vi "AlarmInsert.vi"(6 "提示":string="正常", 7 "takesTime":string, 9 "级别":string="10", 10 "类型":string="装配步骤", 11 "消息名":string) -> ()   [LabVIEW 2013]
uses:
  resultShow.vi
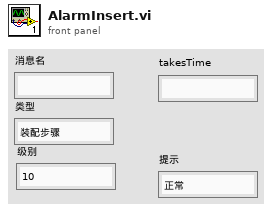
[diagram p1: front panel]
types:
  T1 = cluster{"takesTime":refnum<vi>, "userStatus":refnum<vi>, "userName":refnum<vi>, "connectionMode":refnum<vi>, "productsName":refnum<vi>, "rigStatus":refnum<vi>, "管柱码":refnum<vi>, "上序状态":refnum<vi>}
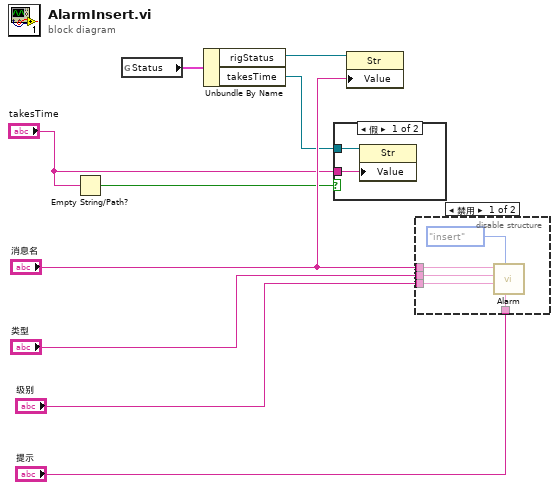
[diagram p0: block diagram]
diagram:
  n1 = Empty String/Path?(string/path="takesTime") -> (empty?=w1:bool)
  n2 = global read "resultShow.vi" "Status"() -> (w9:T1)
  n3 = Unbundle By Name(w9) -> ("rigStatus"=w8:refnum<vi>, "takesTime"=w3:refnum<vi>)
  n4 = case shown="假" w1 {
    tunnel: w3 -> [w11 _]
    tunnel: "takesTime" -> [w10 _]
    frame False {
      n5 = property class="Str"(reference=w11, "Value"=w10) -> ()  [unwired: 1 in, 2 out]
    }
    frame True {
    }
  }
  n6 = property class="Str"(reference=w8, "Value"="消息名") -> ()  [unwired: 1 in, 2 out]
  n7 = disable-structure shown="禁用" {
    disable-tunnel: "类型" -> [w15 _]
    disable-tunnel: "级别" -> [w14 _]
    disable-tunnel: "提示" -> [w13 _]
    disable-tunnel: "消息名" -> [w12 _]
    frame Disabled {
      n8 = call "Alarm.vi"("提示"=w13, "模式"=enum16{"select", "insert", "update", "delete"}."insert", "级别"=w14, "类型"=w15, "消息名"=w12) -> ()  [unwired: 6 in, 1 out]
    }
    frame Enabled {
    }
  }
